vi "Load Shots (SubVI).vi"(3 "Record #":i32, 4 "Method":string) -> (0 "Shot Array":string[][](array[string]), 1 "AvgDef":dbl)   [LabVIEW 2015]
panel:
  in  "error IN":errorcluster
  out "error out":errorcluster
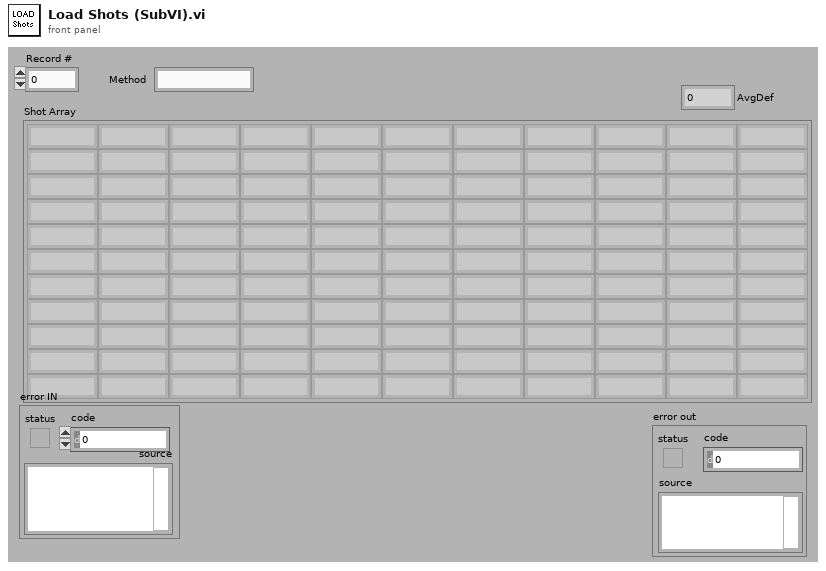
[diagram p1: front panel]
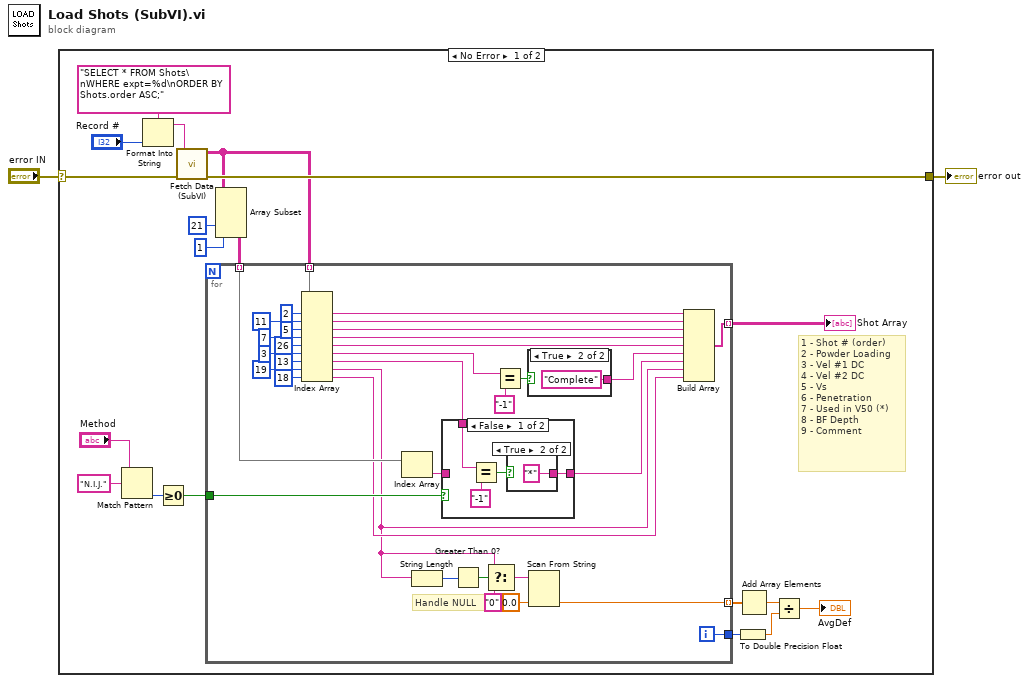
[diagram p0: block diagram]
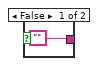
[diagram p2: hidden frame]
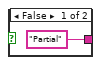
[diagram p4: hidden frame]
diagram:
  n1 = case shown="No Error" "error IN" {
    selector: "error IN" -> [w11 w65]
    tunnel: [w10 w65] -> w1
    frame No Error {
      # "1 - Shot # (order)\n2 - Powder Loading\n3 - Vel #1 DC\n4 - Vel #2 DC\n5 - Vs\n6 - Penetration\n7 - Used in V50 (*)\n8 - BF Depth\n9 - Comment"
      n2 = Match Pattern(string="Method", regular expression="N.I.J.") -> (offset past match=w13:i32)  [unwired: 4 out]
      n3 = Format Into String(format string="SELECT * FROM Shots\nWHERE expt=%d\nORDER BY Shots.order ASC;" ("query string"), "Record #") -> (resulting string=w19:string)  [unwired: 2 in, 1 out]
      n4 = Greater Or Equal To 0?(x=w13) -> (x >= 0?=w12:bool)
      n5 = call "Fetch Data (SubVI).vi"("error IN"=w11, "query string"=w19) -> ("error OUT"=w10:errorcluster, "recordset data"=w9:string[][])  [unwired: 4 out]
      n6 = Array Subset(array=w9, index (col)=21 ("index"), length (col)=1 ("length")) -> (w16:string[][])  [unwired: 2 in]
      n7 = for {
        tunnel: w9 -> [w55] mode=indexing
        tunnel: w16 -> [w52] mode=indexing
        tunnel: w12 -> [w50]
        tunnel: [w47] -> w8 mode=indexing
        tunnel: [w23] -> w7 mode=indexing
        tunnel: [w22] -> w5
        i -> [w22]
        # "Handle NULL"
        n8 = Index Array(array=w55, index #1=2 ("index"), index #2=11 ("index"), index #3=5 ("index"), index #4=7 ("index"), index #5=26 ("index"), index #6=3 ("index"), index #7=13 ("index"), index #8=19 ("index"), index #9=18 ("index")) -> (element #1=w48:string, element #2=w45:string, element #3=w41:string, element #4=w40:string, element #5=w39:string, element #6=w37:string, element #7=w35:string, element #8=w27:string, element #9=w31:string)
        n9 = Index Array(array=w52) -> (element=w51:string)  [unwired: 1 in]
        n10 = String Length(string=w27) -> (length=w29:i32)
        n11 = case shown="False" w50 {
          tunnel: [w59 w62] -> w34
          tunnel: w51 -> [_ w62]
          tunnel: w35 -> [w56 _]
          frame False {
            n12 = Equal?(x=w56, y="-1") -> (x = y?=w57:bool)
            n13 = case shown="True" w57 {
              tunnel: ["" ("Empty String Constant") "*"] -> w59
              frame False {
              }
              frame True {
              }
            }
          }
          frame True {
            # "NIJ Shot Angle"
          }
        }
        n14 = Greater Than 0?(x=w29) -> (x > 0?=w28:bool)
        n15 = Select(t=w27, s=w28, f="0") -> (s? t:f=w25:string)
        n16 = Equal?(x=w37, y="-1") -> (x = y?=w54:bool)
        n17 = case shown="True" w54 {
          tunnel: ["Partial" "Complete"] -> w36
          frame False {
          }
          frame True {
          }
        }
        n18 = Scan From String(input string=w25, default 1=0.0 ("default value 1")) -> (output 1=w23:dbl)  [unwired: 3 in, 3 out]
        n19 = Build Array(w48, w45, w41, w40, w39, w36, w34, w27, w31) -> (w47:string[])
      }
      "Shot Array" <- w8
      n20 = To Double Precision Float(number=w5) -> (double precision float=w4:dbl)
      n21 = Add Array Elements(numeric array=w7) -> (sum=w6:dbl)
      n22 = Divide(x=w6, y=w4) -> (x/y=→"AvgDef":dbl)
    }
    frame Error {
    }
  }
  "error out" <- w1
